vi "Intake Logic.vi"() -> ()   [LabVIEW 2020]
uses:
  <vilib>/Rock Robotics/WPI/ThirdParty/Phoenix-LabVIEW/Motor Controller/Controls/CTRE_Phoenix_MotorControl_ControlMode.ctl
  <vilib>/Rock Robotics/WPI/ThirdParty/REV Robotics/REVLib/Typedef/Spark MAX Control Type.ctl
  <vilib>/Rock Robotics/WPI/Utilities/WPI_GetSetVariantRefNum.vi
  Robot Global Data.vi
  <vilib>/Rock Robotics/Network Tables/NT Read Numeric Array.vi
  2017 Swerve Code/Swerve Global Variables.vi
  <vilib>/addons/control/pid/pid.llb/PID (DBL).vi
  <vilib>/addons/control/pid/NI_PID_pid.lvlib
panel:
  in  "Angle PID 2":T1={"proportional gain (Kc)"=0.03, "integral time (Ti, min)"=0.0, "derivative time (Td, min)"=0.0} {"derivative time (Td, min)" format="%.6f"; "integral time (Ti, min)" format="%.3f"; "proportional gain (Kc)" format="%.3f"}
  in  "output range 2":cluster{"output high":dbl, "output low":dbl}={"output high"=0.5, "output low"=-0.5} {"output low" format="%.2f"; "output high" format="%.2f"}
  in  "Shooter PID":T2={"P Gain"=0.0, "I Gain"=0.0, "D Gain"=0.0, "F Gain"=0.0, "I Zone"=0.0, "Min Output"=-1.0, "Max Output"=1.0}
  in  "Set PID":bool
  in  "speed lookup table":dbl[](array[numeric])
  out "Raspberry pi info":dbl[](array[numeric])
  in  "ball sense voltage":dbl=3.0 format="%#_13g"
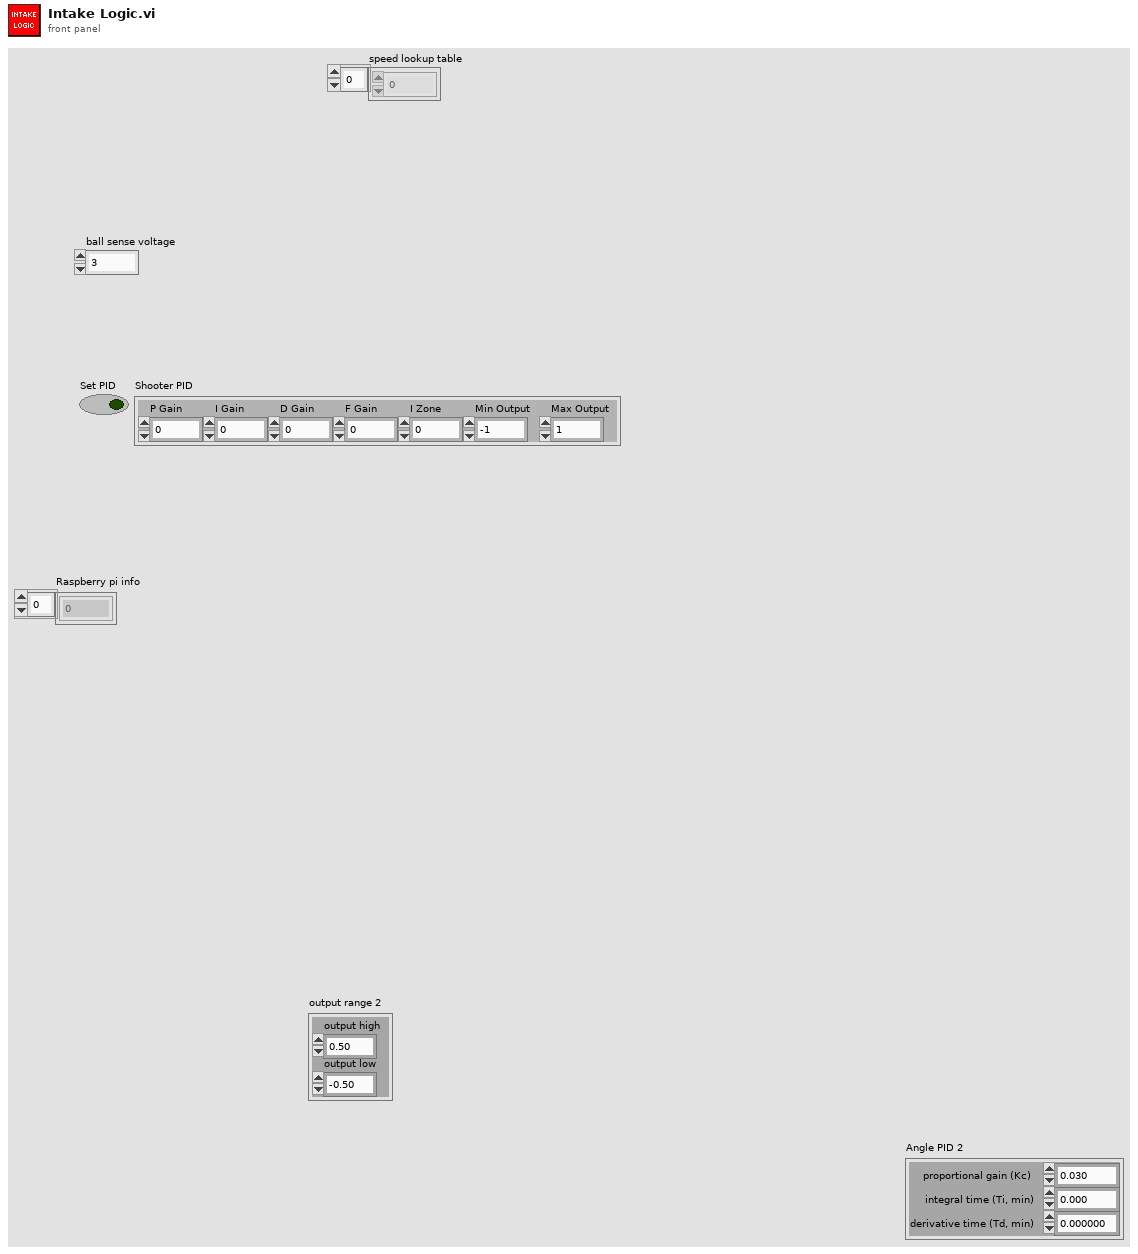
[diagram p1: front panel]
types:
  T1 = cluster{"proportional gain (Kc)":dbl, "integral time (Ti, min)":dbl, "derivative time (Td, min)":dbl}
  T2 = cluster{"P Gain":dbl, "I Gain":dbl, "D Gain":dbl, "F Gain":dbl, "I Zone":dbl, "Min Output":dbl, "Max Output":dbl}
  T3 = typedef "WPI_MotorControlDeviceRef.ctl" = cluster{"DeviceStatus":errorcluster, "Type":T4, "PWM":cluster{"PWM Channel":T5, "DeadBand":T6}, "CAN":cluster{"Device Number":u8, "SetOutput VI Ref":variant, "GetOutput VI Ref":variant, "Enable VI Ref":variant, "Disable VI Ref":variant, "Data":variant}, "Invert":bool, "DIO PWM":cluster{"PWM \"Enable\" Channel":T5, "DIOChannel":T7, "PWM Rate":dbl}}
  T4 = typedef "WPI_MotorControlType.ctl" = enum16{"PWM", "CAN", "DIO PWM"}
  T5 = typedef "FPGA_DIOPWMChannel.ctl" = enum8{"PWM 0", "PWM 1", "PWM 2", "PWM 3", "PWM 4", "PWM 5", "PWM 6", "PWM 7", "PWM 8", "PWM 9", "PWM MXP 0", "PWM MXP 1", "PWM MXP 2", "PWM MXP 3", "PWM MXP 4", "PWM MXP 5", "PWM MXP 6", "PWM MXP 7", "PWM MXP 8", "PWM MXP 9", "Invalid"}
  T6 = typedef "WPI_PWMDeadband.ctl" = cluster{"Name":string, "maxPositivePwm":i32, "minPositivePwm":i32, "centerPwm":i32, "maxNegativePwm":i32, "minNegativePwm":i32, "angularRange":u16}
  T7 = typedef "FPGA_DIOChannel.ctl" = enum8{"DIO 0", "DIO 1", "DIO 2", "DIO 3", "DIO 4", "DIO 5", "DIO 6", "DIO 7", "DIO 8", "DIO 9", "DIO MXP 0", "DIO MXP 1", "DIO MXP 2", "DIO MXP 3", "DIO MXP 4", "DIO MXP 5", "DIO MXP 6", "DIO MXP 7", "DIO MXP 8", "DIO MXP 9", "DIO MXP 10", "DIO MXP 11", "DIO MXP 12", "DIO MXP 13", "DIO MXP 14", "DIO MXP 15", "SPI Port CS1", "SPI Port CS2", "SPI Port CS3", "SPI Port MISO", "SPI Port MOSI", "Invalid"}
  T8 = typedef "WPI_AnalogChannelDevRef.ctl" = cluster{"DevStatus":errorcluster, "Analog Channel":T9}
  T9 = typedef "FPGA_AIChannel.ctl" = enum8{"AI 0", "AI 1", "AI 2", "AI 3", "AI MXP 0", "AI MXP 1", "AI MXP 2", "AI MXP 3", "Invalid"}
  T10 = typedef "Spark MAX Control Type.ctl" = enum16{"Percent VBus", "Voltage", "Velocity", "Position", "Smart Motion", "Current", "Smart Velocity"}
  T11 = typedef "CTRE_Phoenix_MotorControl_ControlMode.ctl" = u16
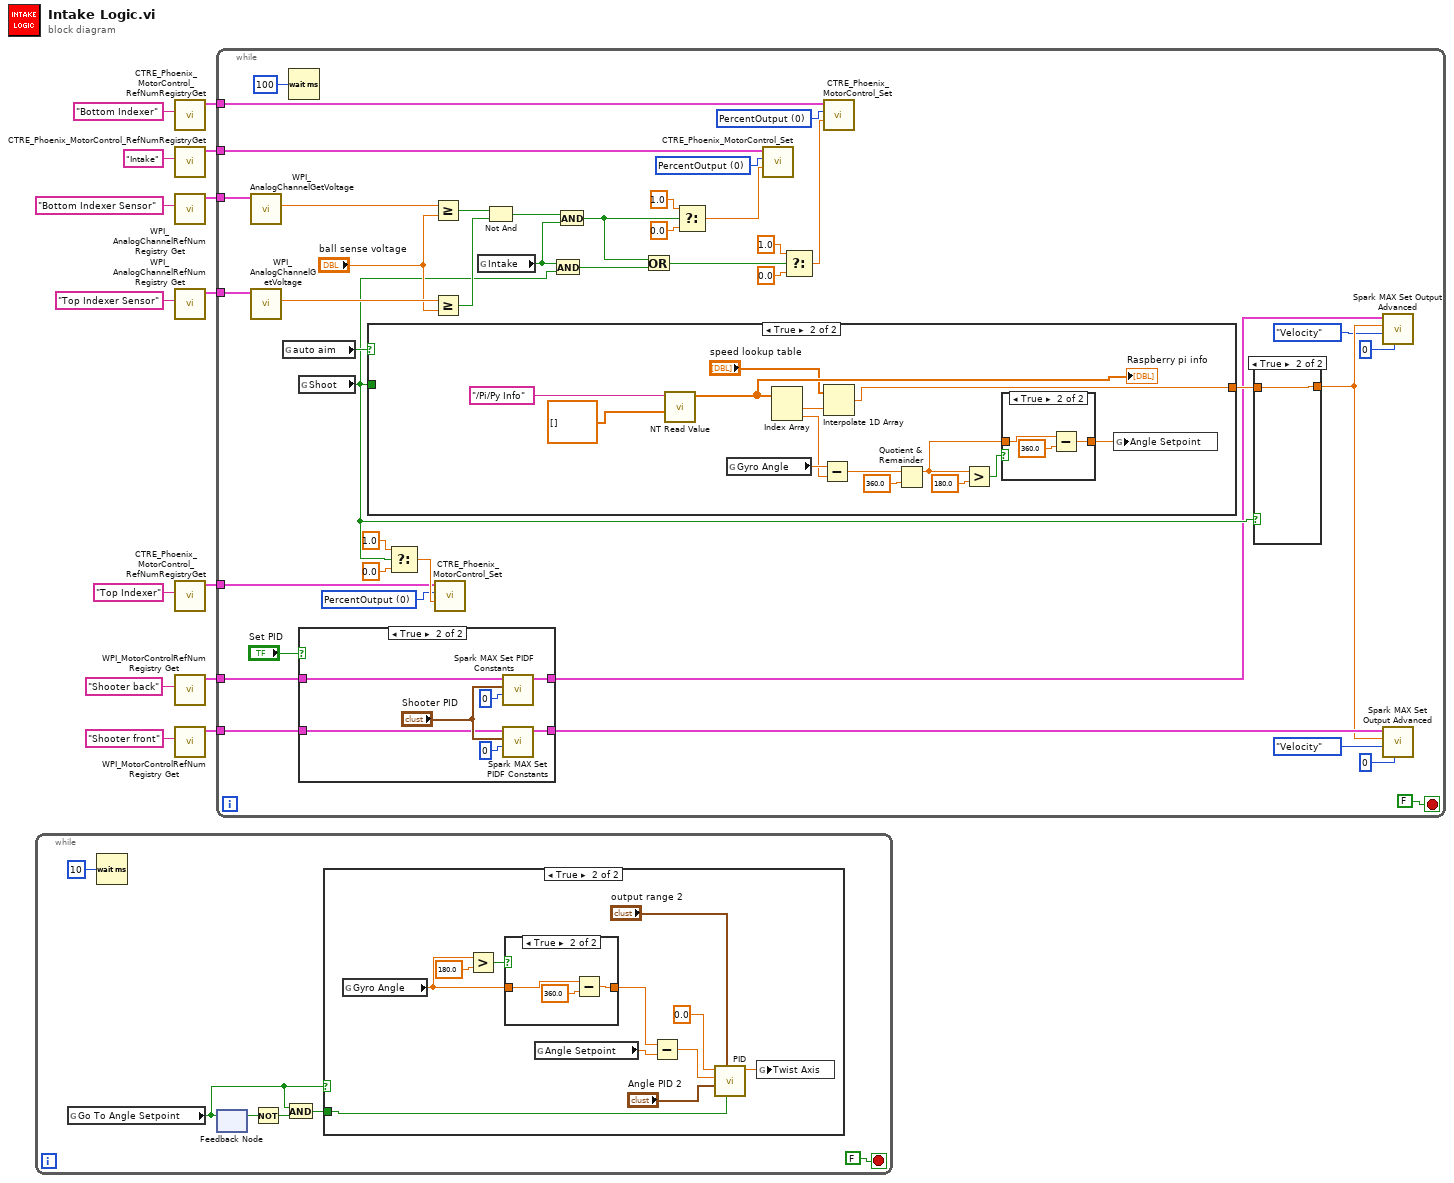
[diagram p0: block diagram]
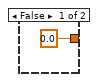
[diagram p4: hidden frame]
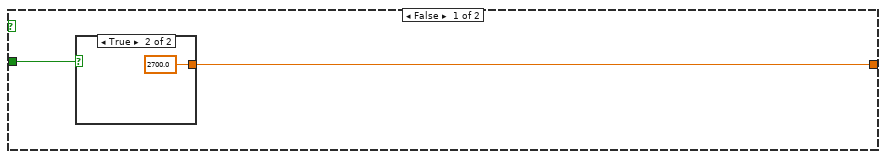
[diagram p6: hidden frame]
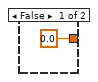
[diagram p7: hidden frame]
diagram:
  n1 = while {
    stop <- FALSE stop-if-true
    n2 = global read "Robot Global Data.vi" "Go To Angle Setpoint"() -> (w16:bool)
    n3 = Wait (ms)(milliseconds to wait=u32 10) -> ()  [unwired: 1 out]
    n4 = feedback-in #1(w16) -> ()
    n5 = feedback #1() -> (w18:bool)  [unwired: 1 in]
    n6 = Not(x=w18) -> (.not. x?=w17:bool)
    n7 = And(x=w16, y=w17) -> (x .and. y?=w15:bool)
    n8 = case shown="True" w16 {
      tunnel: w15 -> [_ w21]
      frame False {
      }
      frame True {
        n9 = global read "Swerve Global Variables.vi" "Gyro Angle"() -> (w25:dbl)
        n10 = Greater?(x=w25, y=180.0) -> (0:w28:bool)
        n11 = case shown="True" w28 {
          tunnel: w25 -> [w32 w34]
          tunnel: [w32 w33] -> w27
          frame False {
          }
          frame True {
            n12 = Subtract(x=w34, y=360.0) -> (x-y=w33:dbl)
          }
        }
        n13 = global read "Robot Global Data.vi" "Angle Setpoint"() -> (w22:dbl)
        n14 = Subtract(x=w27, y=w22) -> (x-y=w30:dbl)
        n15 = call-poly <vilib>:"PID.vi"("reinitialize? (F)"=w21, "output range"="output range 2", "PID gains"="Angle PID 2", "process variable"=w30, "setpoint"=0.0) -> ("output"=w23:dbl)  [unwired: 5 in, 1 out]
        n16 = global write "Swerve Global Variables.vi" "Twist Axis"(w23) -> ()
      }
    }
  }
  n17 = call <vilib>:"CTRE_Phoenix_MotorControl_RefNumRegistryGet.vi"("refnum name"="Bottom Indexer") -> ("PhoenixMotorControlDevRef"=w14:T3)  [unwired: 9 in, 1 out]
  n18 = call <vilib>:"CTRE_Phoenix_MotorControl_RefNumRegistryGet.vi"("refnum name"="Intake") -> ("PhoenixMotorControlDevRef"=w11:T3)  [unwired: 9 in, 1 out]
  n19 = call <vilib>:"WPI_AnalogChannelRefNum Registry Get.vi"("refnum name"="Bottom Indexer Sensor") -> ("AIDeviceRef"=w5:T8)  [unwired: 9 in, 1 out]
  n20 = call <vilib>:"WPI_AnalogChannelRefNum Registry Get.vi"("refnum name"="Top Indexer Sensor") -> ("AIDeviceRef"=w6:T8)  [unwired: 9 in, 1 out]
  n21 = call <vilib>:"CTRE_Phoenix_MotorControl_RefNumRegistryGet.vi"("refnum name"="Top Indexer") -> ("PhoenixMotorControlDevRef"=w9:T3)  [unwired: 9 in, 1 out]
  n22 = call <vilib>:"WPI_MotorControlRefNum Registry Get.vi"("refnum name"="Shooter back") -> ("MotorControlDevRef"=w2:T3)  [unwired: 9 in, 1 out]
  n23 = call <vilib>:"WPI_MotorControlRefNum Registry Get.vi"("refnum name"="Shooter front") -> ("MotorControlDevRef"=w1:T3)  [unwired: 9 in, 1 out]
  n24 = while {
    tunnel: w11 -> [w74]
    tunnel: w14 -> [w75]
    tunnel: w9 -> [w53]
    tunnel: w6 -> [w71]
    tunnel: w5 -> [w70]
    tunnel: w2 -> [w46]
    tunnel: w1 -> [w45]
    stop <- FALSE stop-if-true
    w52 = T11 0 items=["PercentOutput"=0, "Position"=1, "Velocity"=2, "Current"=3, "Follower"=5, "MotionProfile"=6, "MotionMagic"=7, "MotionProfileArc"=10, "Disabled"=15] ("Control Mode")
    w72 = T11 0 items=["PercentOutput"=0, "Position"=1, "Velocity"=2, "Current"=3, "Follower"=5, "MotionProfile"=6, "MotionMagic"=7, "MotionProfileArc"=10, "Disabled"=15] ("Control Mode")
    w73 = T11 0 items=["PercentOutput"=0, "Position"=1, "Velocity"=2, "Current"=3, "Follower"=5, "MotionProfile"=6, "MotionMagic"=7, "MotionProfileArc"=10, "Disabled"=15] ("Control Mode")
    n25 = call <vilib>:"WPI_AnalogChannelGetVoltage.vi"("AIDeviceRef"=w70) -> ("Voltage"=w69:dbl)  [unwired: 8 in, 2 out]
    n26 = call <vilib>:"WPI_AnalogChannelGetVoltage.vi"("AIDeviceRef"=w71) -> ("Voltage"=w68:dbl)  [unwired: 8 in, 2 out]
    n27 = global read "Robot Global Data.vi" "auto aim"() -> (w48:bool)
    n28 = Wait (ms)(milliseconds to wait=u32 100) -> ()  [unwired: 1 out]
    n29 = global read "Robot Global Data.vi" "Shoot"() -> (w43:bool)
    n30 = case shown="True" "Set PID" {
      tunnel: w46 -> [w81 w87]
      tunnel: w45 -> [w80 w86]
      tunnel: [w80 w83] -> w41
      tunnel: [w81 w82] -> w42
      frame False {
      }
      frame True {
        n31 = call <vilib>:"Spark MAX Set PIDF Constants.vi"("PIDF Slot"=0, "PID Constants"="Shooter PID", "MotorControlDeviceRef"=w87) -> ("MotorControlDeviceRef"=w82:T3)  [unwired: 7 in, 1 out]
        n32 = call <vilib>:"Spark MAX Set PIDF Constants.vi"("PIDF Slot"=0, "PID Constants"="Shooter PID", "MotorControlDeviceRef"=w86) -> ("MotorControlDeviceRef"=w83:T3)  [unwired: 7 in, 1 out]
      }
    }
    n33 = case shown="True" w48 {
      tunnel: [w89 w101] -> w44
      tunnel: w43 -> [w90 _]
      frame False {
        n34 = case shown="True" w90 {
          tunnel: [0.0 2700.0] -> w89
          frame False {
          }
          frame True {
          }
        }
      }
      frame True {
        n35 = call-poly <vilib>:"NT Read Value.vi"("Default Value"=dbl[] [], "Name"="/Pi/Py Info") -> ("Numeric Array"=w104:dbl[])  [unwired: 8 in, 1 out]
        "Raspberry pi info" <- w104
        n36 = global read "Swerve Global Variables.vi" "Gyro Angle"() -> (w100:dbl)
        n37 = Index Array(array=w104) -> (element #1=w102:dbl, element #2=w93:dbl)  [unwired: 2 in]
        n38 = Subtract(x=w100, y=w93) -> (x-y=w99:dbl)
        n39 = Interpolate 1D Array(1:w102, 2:"speed lookup table") -> (0:w101:dbl)
        n40 = Quotient & Remainder(x=w99, y=360.0) -> (x-y*floor(x/y)=w95:dbl)  [unwired: 1 out]
        n41 = Greater?(x=w95, y=180.0) -> (0:w96:bool)
        n42 = case shown="True" w96 {
          tunnel: [w107 w108] -> w94
          tunnel: w95 -> [w107 w110]
          frame False {
          }
          frame True {
            n43 = Subtract(x=w110, y=360.0) -> (x-y=w108:dbl)
          }
        }
        n44 = global write "Robot Global Data.vi" "Angle Setpoint"(w94) -> ()
      }
    }
    n45 = Select(t=1.0, s=w43, f=0.0) -> (s? t:f=w54:dbl)
    n46 = Greater Or Equal?(x=w69, y="ball sense voltage") -> (x >= y?=w65:bool)
    n47 = Greater Or Equal?(x=w68, y="ball sense voltage") -> (x >= y?=w66:bool)
    n48 = call <vilib>:"CTRE_Phoenix_MotorControl_Set.vi"("Output"=w54, "Control Mode"=w52, "PhoenixMotorControlDevRef"=w53) -> ()  [unwired: 7 in, 2 out]
    n49 = global read "Robot Global Data.vi" "Intake"() -> (w50:bool)
    n50 = Not And(1:w66, 2:w65) -> (0:w49:bool)
    n51 = And(x=w50, y=w43) -> (x .and. y?=w58:bool)
    n52 = And(x=w49, y=w50) -> (x .and. y?=w51:bool)
    n53 = Or(x=w51, y=w58) -> (x .or. y?=w57:bool)
    n54 = Select(t=1.0, s=w51, f=0.0) -> (s? t:f=w56:dbl)
    n55 = call <vilib>:"CTRE_Phoenix_MotorControl_Set.vi"("Output"=w56, "Control Mode"=w73, "PhoenixMotorControlDevRef"=w74) -> ()  [unwired: 7 in, 2 out]
    n56 = Select(t=1.0, s=w57, f=0.0) -> (s? t:f=w55:dbl)
    n57 = call <vilib>:"CTRE_Phoenix_MotorControl_Set.vi"("Output"=w55, "Control Mode"=w72, "PhoenixMotorControlDevRef"=w75) -> ()  [unwired: 7 in, 2 out]
    n58 = case shown="True" w43 {
      tunnel: [0.0 w79] -> w40
      tunnel: w44 -> [_ w79]
      frame False {
      }
      frame True {
      }
    }
    n59 = call <vilib>:"Spark MAX Set Output Advanced.vi"("PIDF Slot (0)"=0, "Control Mode"=Spark_MAX_Control_Type."Velocity", "Setpoint"=w40, "MotorControlDevRef"=w42) -> ()  [unwired: 6 in, 2 out]
    n60 = call <vilib>:"Spark MAX Set Output Advanced.vi"("PIDF Slot (0)"=0, "Control Mode"=Spark_MAX_Control_Type."Velocity", "Setpoint"=w40, "MotorControlDevRef"=w41) -> ()  [unwired: 6 in, 2 out]
  }
